vi "open_powermeter-v2.vi"(11 "VISA Refnum in":refnum<visa-resource-name>) -> (0 "error out":errorcluster)   [LabVIEW 2021]
doc: "André Romero - 2024\nandretec@ifsc.usp.br"
uses:
  Global_v20.vi
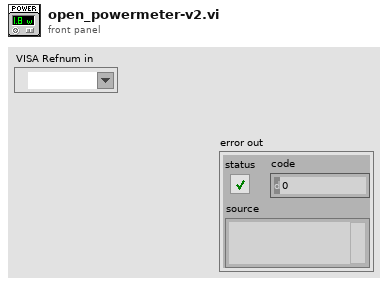
[diagram p1: front panel]
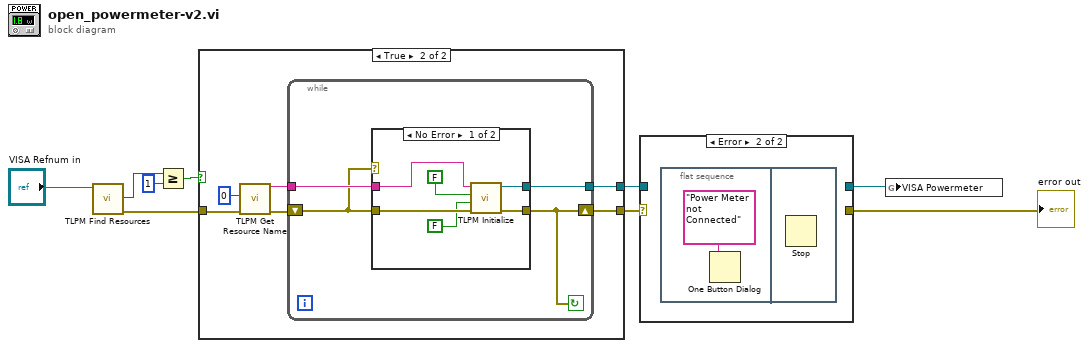
[diagram p0: block diagram]
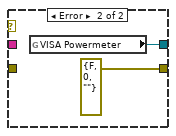
[diagram p3: hidden frame]
diagram:
  n1 = call <instrlib>:"TLPM Find Resources.vi"("instrument handle"="VISA Refnum in") -> ("error out"=w6:errorcluster, "Resource Count"=w3:u32)  [unwired: 8 in, 1 out]
  n2 = Greater Or Equal?(x=w3, y=u32 1) -> (x >= y?=w5:bool)
  n3 = case shown="True" w5 {
    tunnel: [_ w13] -> w8
    tunnel: [w10 w12] -> w7
    tunnel: w6 -> [w10 w11]
    frame False {
    }
    frame True {
      n4 = call <instrlib>:"TLPM Get Resource Name.vi"("error in (no error)"=w11, "Index (0)"=u32 0 ("Device Index")) -> ("error out"=w16:errorcluster, "Resource Name"=w15:string)  [unwired: 7 in, 1 out]
      n5 = while {
        tunnel: w15 -> [w20]
        tunnel: [w19] -> w13
        shift-right: [w18] -> w12
        shift-left: w16 -> [w17]
        stop <- w18 continue-if-true
        n6 = case shown="No Error" w17 {
          tunnel: w17 -> [w26 _]
          tunnel: w20 -> [w25 _]
          tunnel: [w23 w28] -> w19
          tunnel: [w22 errorcluster {"status"=FALSE, "code"=0, "source"=""} ("error out")] -> w18
          frame No Error {
            n7 = call <instrlib>:"TLPM Initialize.vi"("error in (no error)"=w26, "Reset Device (Reset Device)"=FALSE, "ID Query (Do Query)"=FALSE, "resource name"=w25) -> ("error out"=w22:errorcluster, "instrument handle out"=w23:refnum<visa-resource-name>)  [unwired: 6 in]
          }
          frame Error {
            n8 = global read "Global_v20.vi" "VISA Powermeter"() -> (w28:refnum<visa-resource-name>)
          }
        }
      }
    }
  }
  n9 = case shown="Error" w7 {
    selector: w7 -> [w29 _]
    tunnel: w8 -> [w30 _]
    tunnel: [w30 _] -> w9
    tunnel: [w29 _] -> w1
    frame No Error {
    }
    frame Error {
      n10 = flat-sequence {
        frame #0 {
          n11 = One Button Dialog(message="Power Meter not Connected") -> ()  [unwired: 1 in, 1 out]
        }
        frame #1 {
          n12 = Stop() -> ()  [unwired: 1 in]
        }
      }
    }
  }
  "error out" <- w1
  n13 = global write "Global_v20.vi" "VISA Powermeter"(w9) -> ()
